vi "FullScreen.vi"(11 "VIRef":refnum<vi>) -> (3 "output cluster":T1)   [LabVIEW 2021]
doc: "使VI全屏显示。\n20140516\n蒋松。"
uses:
  <vilib>/Utility/miscctls.llb/LVRectTypeDef.ctl
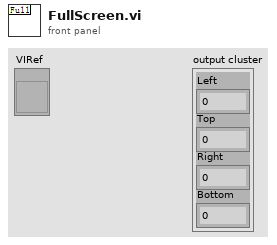
[diagram p1: front panel]
types:
  T1 = typedef "LVRectTypeDef.ctl" = cluster{"Left":i16, "Top":i16, "Right":i16, "Bottom":i16}
  T2 = typedef "LVAllMonitorsDisplayTypeDef.ctl" = cluster{"Bounds":cluster{"Left":i16, "Top":i16, "Right":i16, "Bottom":i16}, "Depth":i16}[]
  T3 = cluster{"Bounds":cluster{"Left":i16, "Top":i16, "Right":i16, "Bottom":i16}, "Depth":i16}
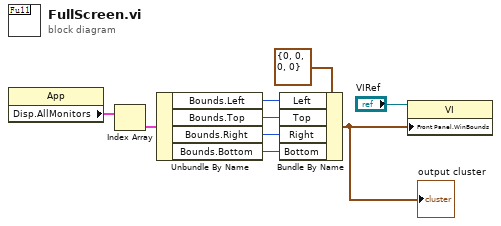
[diagram p0: block diagram]
diagram:
  n1 = property class="App"() -> ("Disp.AllMonitors"=w9:T2)  [unwired: 2 in, 2 out]
  n2 = Index Array(array=w9) -> (element=w8:T3)  [unwired: 1 in]
  n3 = Unbundle By Name(w8) -> ("Bounds.Left"=w6:i16, "Bounds.Top"=w4:i16, "Bounds.Right"=w3:i16, "Bounds.Bottom"=w2:i16)
  n4 = Bundle By Name(cluster=T1 {"Left"=0, "Top"=0, "Right"=0, "Bottom"=0} ("Front Panel Window:Window Bounds"), "Left"=w6, "Top"=w4, "Right"=w3, "Bottom"=w2) -> (w5:T1)
  "output cluster" <- w5
  n5 = property class="VI"(reference="VIRef", "Front Panel.WinBounds"=w5) -> ()  [unwired: 1 in, 2 out]
